vi "ImageReadImage-1D.vi"(8 "error in (no error)":errorcluster, 11 "Image in":refnum<class "Image.lvclass">) -> (0 "error out":errorcluster, 2 "Images":dbl[][][](array[numeric]), 3 "Image out":refnum<class "Image.lvclass">)   [LabVIEW 2012, in "Image.lvclass"]
uses:
  classes/Image.lvclass
  classes/Image.lvclass/Image.ctl
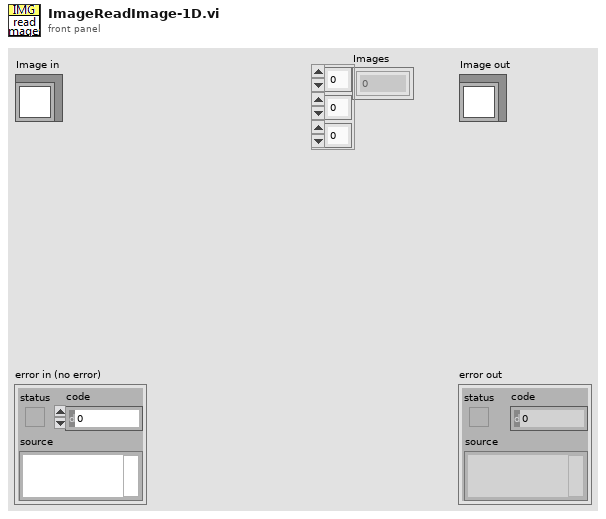
[diagram p1: front panel]
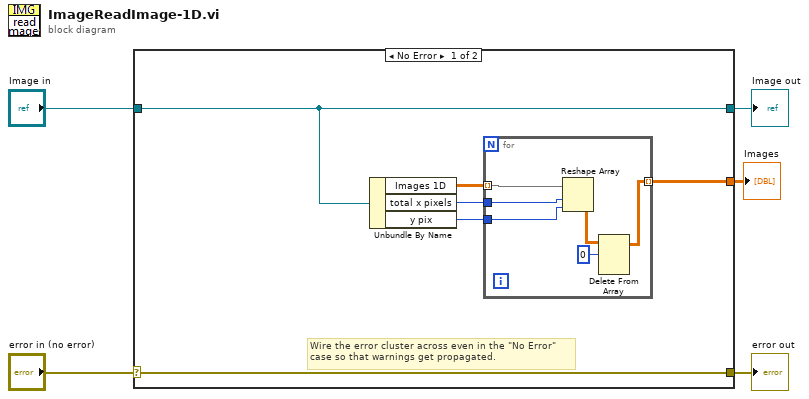
[diagram p0: block diagram]
diagram:
  n1 = case shown="No Error" "error in (no error)" {
    selector: "error in (no error)" -> [w11 w19]
    tunnel: [w11 w19] -> w4
    tunnel: [w10 w18] -> w2
    tunnel: "Image in" -> [w10 w18]
    tunnel: [w6 _] -> w1
    frame No Error {
      # "Wire the error cluster across even in the \"No Error\"\ncase so that warnings get propagated."
      n2 = Unbundle By Name(w10) -> ("Images 1D"=w9:dbl[][][], "total x pixels"=w8:i32, "y pix"=w7:i32)
      n3 = for {
        tunnel: w9 -> [w17] mode=indexing
        tunnel: w8 -> [w16]
        tunnel: w7 -> [w15]
        tunnel: [w13] -> w6 mode=indexing
        n4 = Reshape Array(w17, w16, w15) -> (w14:dbl[][])
        n5 = Delete From Array(array=w14, length=0) -> (array with subset deleted=w13:dbl[][])  [unwired: 2 in, 1 out]
      }
    }
    frame Error {
    }
  }
  "error out" <- w4
  "Image out" <- w2
  "Images" <- w1
